vi "Get Arc Velocity from Wheels.vi"(5 "wheel indexes":i32[](array[numeric]), 6 "constraint error tolerance (1E-12)":dbl=1e-12, 7 "get motor data (F)":bool, 8 "error in (no error)":errorcluster, 9 "acquired wheel states":T1[](array[typedef]), 11 "steering frame in":refnum<class "NI_Robotics_Steering Frame.lvclass">) -> (0 "error out":errorcluster, 1 "wheel states":T1[](array[typedef]), 2 "estimated arc velocity":T2={"turning radius"=1.0, "tangential velocity"=0.0, "angle from tangent (rad)"=0.0}, 3 "steering frame out":refnum<class "NI_Robotics_Steering Frame.lvclass">)   [LabVIEW 2017, in "NI_Robotics_Steering Frame.lvclass"]
doc: "Calculates the steering frame velocity or arc velocity required to best satisfy the state of each wheel. You can read data for each wheel from wheel motors or specify the wheel data manually. You must manually select the polymorphic instance to use."
uses:
  <vilib>/robotics/Steering/Steering Frame/NI_Robotics_Steering Frame.lvclass
  <vilib>/robotics/Steering/Wheel/Wheel State.ctl
  <vilib>/robotics/Steering/Steering Frame/Arc Velocity.ctl
  <vilib>/robotics/Steering/Wheel/NI_Robotics_Wheel.lvclass
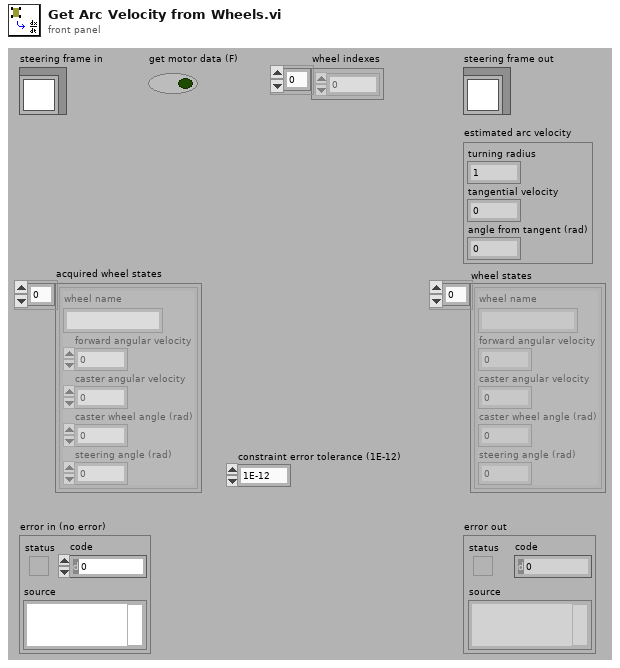
[diagram p1: front panel]
types:
  T1 = typedef "NI_Robotics_Wheel.lvclass/Wheel State.ctl" = cluster{"wheel name":string, "forward angular velocity":dbl, "caster angular velocity":dbl, "caster wheel angle (rad)":dbl, "steering angle (rad)":dbl}
  T2 = typedef "NI_Robotics_Steering Frame.lvclass/Arc Velocity.ctl" = cluster{"turning radius":dbl, "tangential velocity":dbl, "angle from tangent (rad)":dbl}
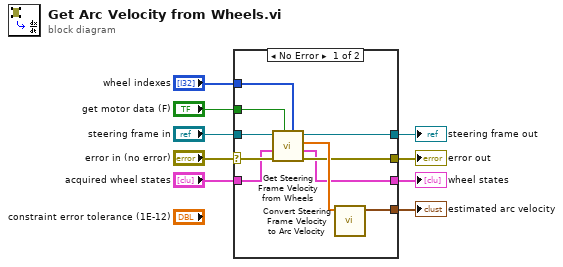
[diagram p0: block diagram]
diagram:
  n1 = case shown="No Error" "error in (no error)" {
    selector: "error in (no error)" -> [w16 w22]
    tunnel: [w13 w22] -> w8
    tunnel: [w18 w21] -> w6
    tunnel: "steering frame in" -> [w19 w21]
    tunnel: "get motor data (F)" -> [w17 _]
    tunnel: "acquired wheel states" -> [w15 w20]
    tunnel: [w12 _] -> w3
    tunnel: [w11 w20] -> w2
    tunnel: "wheel indexes" -> [w10 _]
    frame No Error {
      n2 = call <vilib>:"Get Steering Frame Velocity from Wheels.vi"("wheel indexes"=w10, "get motor data (F)"=w17, "error in (no error)"=w16, "acquired wheel states"=w15, "steering frame in"=w19) -> ("error out"=w13:errorcluster, "wheel states"=w11:T1[], "estimated steering frame velocity"=w14:dbl[], "steering frame out"=w18:refnum<class "NI_Robotics_Steering Frame.lvclass">)  [unwired: 3 in]
      n3 = call <vilib>:"Convert Steering Frame Velocity to Arc Velocity.vi"("steering frame velocity"=w14) -> ("arc velocity"=w12:T2)  [unwired: 10 in]
    }
    frame Error {
    }
  }
  "error out" <- w8
  "steering frame out" <- w6
  "estimated arc velocity" <- w3
  "wheel states" <- w2
